vi "Create Folder.vi"(8 "error in":errorcluster, 11 "Report in":refnum<class "Report.lvclass">) -> (0 "error out":errorcluster, 3 "Report out":refnum<class "Report.lvclass">)   [LabVIEW 2023, in "Report.lvlib" / "Report.lvclass"]
uses:
  Report.lvclass
  Report.lvclass/Report.ctl
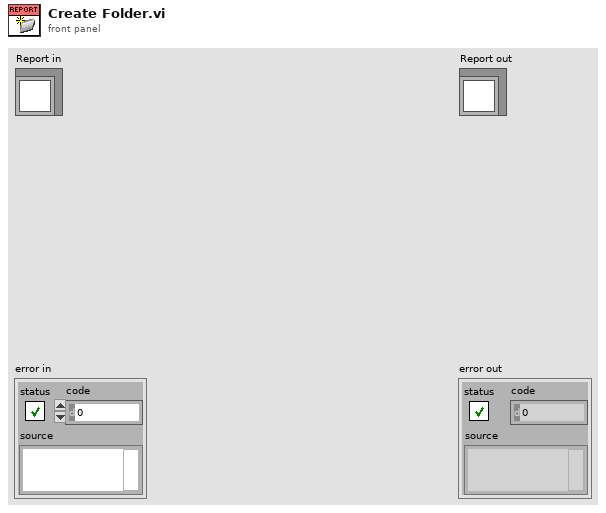
[diagram p1: front panel]
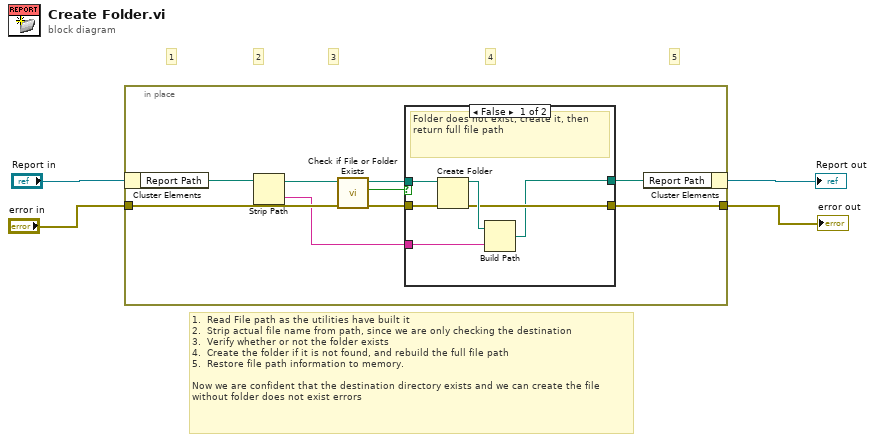
[diagram p0: block diagram]
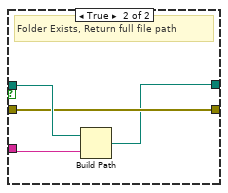
[diagram p2: hidden frame]
diagram:
  # "1.  Read File path as the utilities have built it\n2.  Strip actual file name from path, since we are only checking the destination\n3.  Verify whether or not the folder exists\n4.  Create the folder if it is not found, and rebuild the full file path\n5.  Restore file path information to memory.  \n\nNow we are confident that the destination directory exists and we can create the file\nwithout folder does not exist errors"
  # "5"
  # "4"
  # "3"
  # "2"
  # "1"
  n1 = in-place {
    in-place-border: "error in" -> [w13]
    in-place-border: [w7] -> w3
    n2 = in-place-cluster #1("Report in") -> ("Report Path"=w6:path)
    n3 = Strip Path(path=w6) -> (stripped path=w9:path, name=w8:string)
    n4 = call <vilib>:"Check if File or Folder Exists.vi"("error in (no error)"=w13, "path"=w9) -> ("error out"=w11:errorcluster, "file or folder exists?"=w12:bool, "dup path"=w10:path)  [unwired: 7 in]
    n5 = case shown="False" w12 {
      tunnel: w11 -> [w19 w21]
      tunnel: w10 -> [w18 w22]
      tunnel: w8 -> [w16 w23]
      tunnel: [w15 w21] -> w7
      tunnel: [w14 w20] -> w5
      frame False {
        # "Folder does not exist, create it, then return full file path"
        n6 = Create Folder(path (use dialog)=w18, error in=w19) -> (created path=w17:path, error out=w15:errorcluster)  [unwired: 1 in, 1 out]
        n7 = Build Path(base path=w17, name or relative path=w16) -> (appended path=w14:path)
      }
      frame True {
        # "Folder Exists, Return full file path"
        n8 = Build Path(base path=w22, name or relative path=w23) -> (appended path=w20:path)
      }
    }
    n9 = in-place-cluster #1("Report Path"=w5) -> (→"Report out":refnum<class "Report.lvclass">)
  }
  "error out" <- w3
